vi "Show Window.vi"(8 "error in (no error)":errorcluster, 10 "Window State":u32, 11 "hwnd":u32) -> (0 "error out":errorcluster, 3 "Wnd previously Visible?":u32)   [LabVIEW 2016, in "LV MDI.lvclass"]
doc: "Set Window State.(Window Hide-0,Window Display-5)"
uses:
  LV MDI.lvclass
  user32.dll
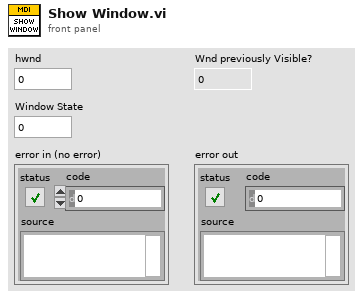
[diagram p1: front panel]
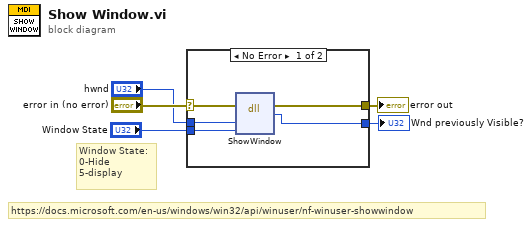
[diagram p0: block diagram]
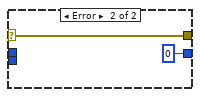
[diagram p2: hidden frame]
diagram:
  # "https://docs.microsoft.com/en-us/windows/win32/api/winuser/nf-winuser-showwindow"
  # "Window State:\n0-Hide\n5-display"
  n1 = case shown="No Error" "error in (no error)" {
    selector: "error in (no error)" -> [w10 w12]
    tunnel: "hwnd" -> [w9 _]
    tunnel: [w8 u32 0 ("bool")] -> w3
    tunnel: [w7 w12] -> w2
    tunnel: "Window State" -> [w6 _]
    frame No Error {
      n2 = dll-call lib="user32.dll" fn="ShowWindow"(error in=w10, "hwnd"=w9, "nCmdShow"=w6) -> (error out=w7:errorcluster, "bool"=w8:u32)  [unwired: 4 in, 1 out]
    }
    frame Error {
    }
  }
  "Wnd previously Visible?" <- w3
  "error out" <- w2
